vi "test-30frame-QR-static.vi"() -> ()   [LabVIEW 2015]
panel:
  in  "stop":bool
  out "data-gobal":string
  out "sum package":dbl
  out "Found?":bool
  out "Mass (kg):":dbl
  out "Style":string
  out "Tong K/lg (kg)":dbl
  out "Quantity":i32
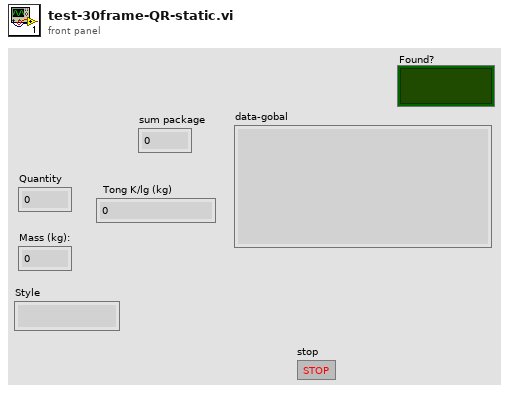
[diagram p1: front panel]
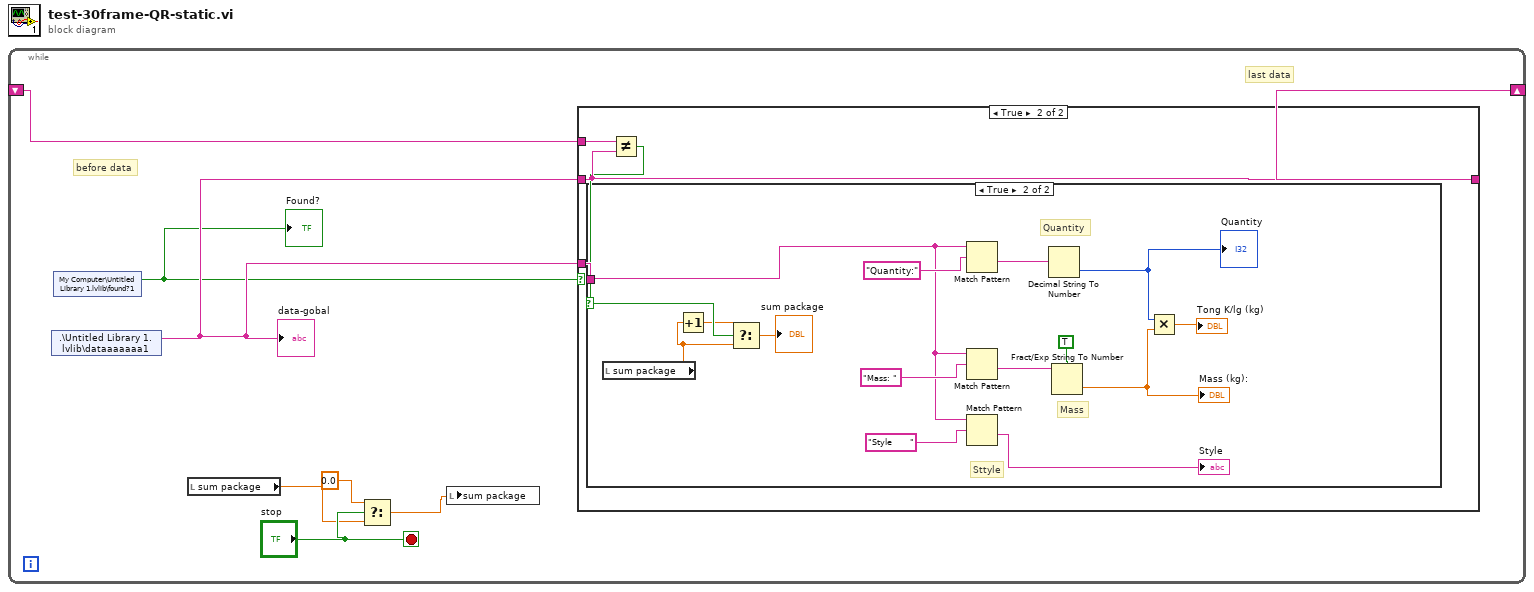
[diagram p0: block diagram]
diagram:
  n1 = while {
    shift-right: [w8] -> _
    shift-left: _ -> [w7]
    stop <- "stop" stop-if-true
    # "before data"
    # "last data"
    n2 = shared-variable ".\\Untitled Library 1.lvlib\\dataaaaaaa1"() -> (w6:string)  [unwired: 1 in, 1 out]
    "data-gobal" <- w6
    n3 = shared-variable "My Computer\\Untitled Library 1.lvlib\\found?1"() -> (w5:bool)  [unwired: 1 in, 1 out]
    "Found?" <- w5
    n4 = local read "sum package"() -> (w1:dbl)
    n5 = Select(t=0.0, s="stop", f=w1) -> (s? t:f=w3:dbl)
    n6 = local write "sum package"(w3) -> ()
    n7 = case shown="True" w5 {
      tunnel: w6 -> [_ w13]
      tunnel: [w9 w11] -> w8
      tunnel: w7 -> [w9 w12]
      tunnel: w6 -> [_ w11]
      frame False {
      }
      frame True {
        n8 = Not Equal?(x=w12, y=w11) -> (x != y?=w10:bool)
        n9 = case shown="True" w10 {
          selector: w10 -> [_ w17]
          tunnel: w13 -> [_ w18]
          frame False {
          }
          frame True {
            # "Sttyle"
            # "Mass"
            # "Quantity"
            n10 = local read "sum package"() -> (w15:dbl)
            n11 = Increment(x=w15) -> (x+1=w16:dbl)
            n12 = Select(t=w16, s=w17, f=w15) -> (s? t:f=→"sum package":dbl)
            n13 = Match Pattern(string=w18, regular expression="Quantity:") -> (after substring=w28:string)  [unwired: 1 in, 3 out]
            n14 = Match Pattern(string=w18, regular expression="Mass: ") -> (after substring=w26:string)  [unwired: 1 in, 3 out]
            n15 = Match Pattern(string=w18, regular expression="Style      ") -> (after substring=→"Style":string)  [unwired: 1 in, 3 out]
            n16 = Decimal String To Number(string=w28) -> (number=w21:i32)  [unwired: 2 in, 1 out]
            "Quantity" <- w21
            n17 = Fract/Exp String To Number(use system decimal point (T)=TRUE, string=w26) -> (number=w20:dbl)  [unwired: 2 in, 1 out]
            "Mass (kg):" <- w20
            n18 = Multiply(x=w21, y=w20) -> (x*y=→"Tong K/lg (kg)":dbl)
          }
        }
      }
    }
  }
